vi "Single channel reverb.vi"(8 "tail length":i32, 9 "fade gain":dbl, 10 "fade delay":i32, 11 "data in":waveform(dbl)) -> (3 "data out":waveform(dbl))   [LabVIEW 2023]
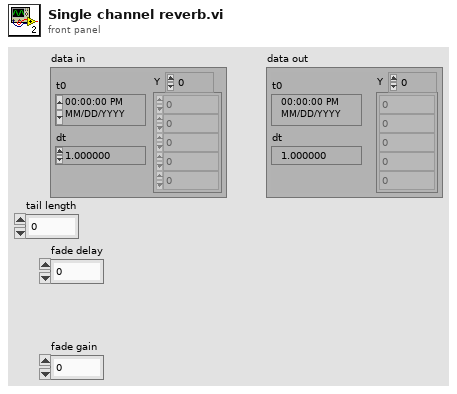
[diagram p1: front panel]
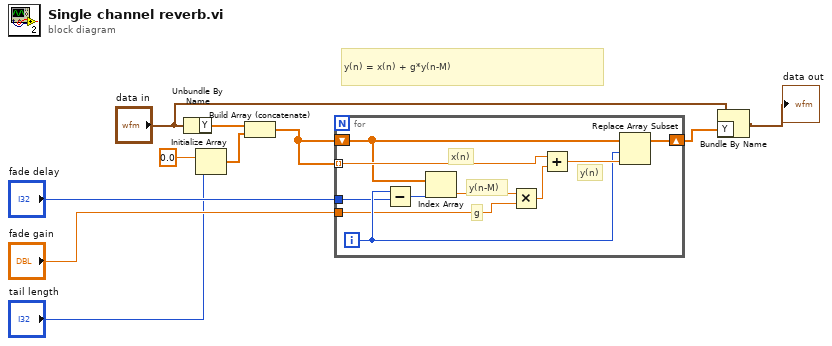
[diagram p0: block diagram]
diagram:
  # "y(n) = x(n) + g*y(n-M)"
  n1 = Unbundle By Name("data in") -> ("Y"=w7:dbl[])
  n2 = Initialize Array(0.0 ("element"), "tail length") -> (w3:dbl[])
  n3 = Build Array (concatenate)(w7, w3) -> (w4:dbl[])
  n4 = for {
    tunnel: w4 -> [w18] mode=indexing
    shift-right: [w20] -> w8
    shift-left: w4 -> [w11]
    tunnel: "fade delay" -> [w14]
    tunnel: "fade gain" -> [w12]
    i -> [w17]
    # "y(n)"
    # "x(n)"
    # "y(n-M)"
    # "g"
    n5 = Subtract(x=w17, y=w14) -> (x-y=w15:i32)
    n6 = Index Array(array=w11, index=w15) -> (element=w16:dbl)
    n7 = Multiply(x=w16, y=w12) -> (x*y=w13:dbl)
    n8 = Add(x=w18, y=w13) -> (x+y=w19:dbl)
    n9 = Replace Array Subset(array=w11, new element=w19, index=w17) -> (w20:dbl[])
  }
  n10 = Bundle By Name(cluster="data in", "Y"=w8) -> (→"data out":waveform(dbl))
